vi "CheckForAutoLogout.vi"() -> (3 "Boolean":bool)   [LabVIEW 2019]
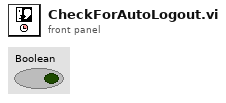
[diagram p1: front panel]
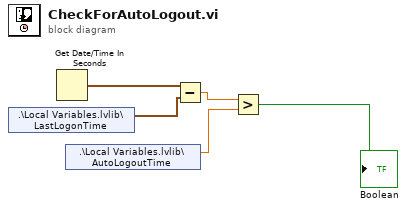
[diagram p0: block diagram]
diagram:
  n1 = shared-variable ".\\Local Variables.lvlib\\LastLogonTime"() -> (w2:timestamp)  [unwired: 1 in, 1 out]
  n2 = Get Date/Time In Seconds() -> (seconds since 1Jan1904=w1:timestamp)
  n3 = shared-variable ".\\Local Variables.lvlib\\AutoLogoutTime"() -> (w4:dbl)  [unwired: 1 in, 1 out]
  n4 = Subtract(x=w1, y=w2) -> (x-y=w3:dbl)
  n5 = Greater?(x=w3, y=w4) -> (0:→"Boolean":bool)
